vi "get_setpoint.vi"(0 "VISA resource name":refnum<visa-resource-name>, 11 "error in (no error)":errorcluster) -> (4 "VISA resource name out":refnum<visa-resource-name>, 13 "Current Setpoint / K":dbl format="%.5f", 15 "error out":errorcluster)   [LabVIEW 2023]
uses:
  <instrlib>/Lake Shore 336/Lake Shore 336.lvlib
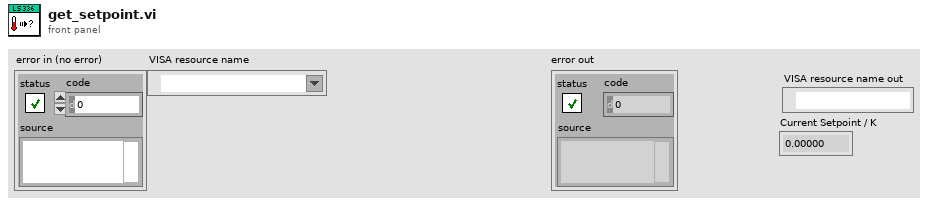
[diagram p1: front panel]
types:
  T1 = cluster{"Baud Rate":u32, "Parity":u16, "Data Bits":u16, "Stop Bits":u16, "Flow Control":u16}
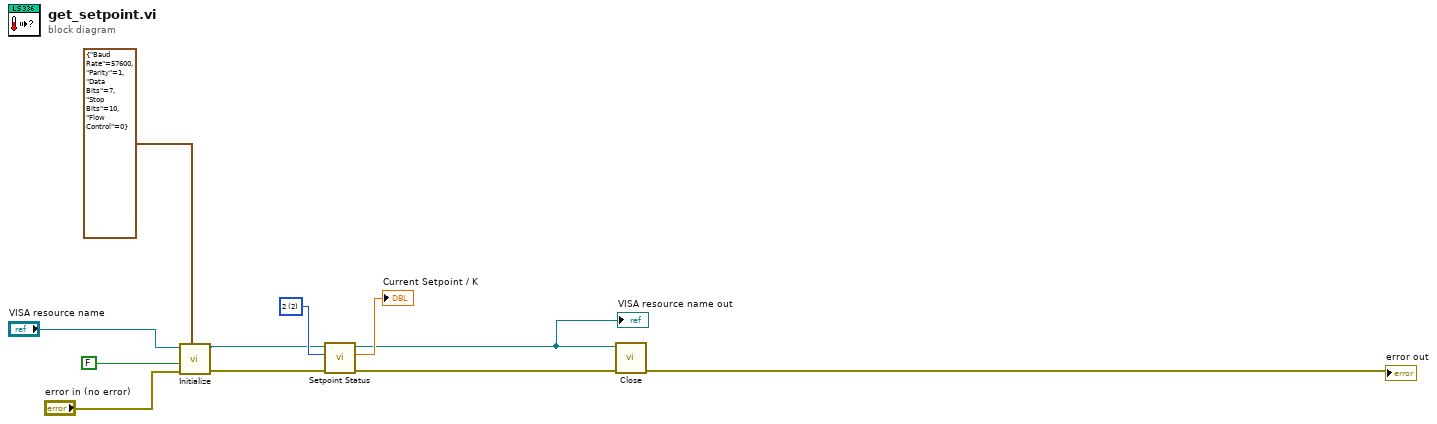
[diagram p0: block diagram]
diagram:
  w6 = u16 2 items=["1"=1, "2"=2, "3"=3, "4"=4] ("Output (1:1)")
  n1 = call <instrlib>:"Initialize.vi"("Serial Configuration"=T1 {"Baud Rate"=57600, "Parity"=1, "Data Bits"=7, "Stop Bits"=10, "Flow Control"=0}, "error in (no error)"="error in (no error)", "Reset (True)"=FALSE, "VISA resource name"="VISA resource name") -> ("error out"=w3:errorcluster, "VISA resource name out"=w4:refnum<visa-resource-name>)  [unwired: 6 in]
  n2 = call <instrlib>:"Setpoint Status.vi"("error in (no error)"=w3, "Output (1:1)"=w6, "VISA resource name"=w4) -> ("error out"=w2:errorcluster, "Setpoint"=→"Current Setpoint / K":dbl, "VISA resource name out"=w1:refnum<visa-resource-name>)  [unwired: 6 in]
  "VISA resource name out" <- w1
  n3 = call <instrlib>:"Close.vi"("error in (no error)"=w2, "VISA resource name"=w1) -> ("error out"=→"error out":errorcluster)  [unwired: 9 in]
